vi "Configure Modulation (Frequency).vi"(4 "Peak Deviation (100.00 Hz)":dbl=100.0, 6 "Modulation Frequency (10 Hz)":dbl=10.0, 7 "Enable Frequency Modulation (T:Enable)":bool=TRUE, 8 "error in (no error)":errorcluster, 9 "Modulation Waveform (Sine)":T1(ring), 10 "FM Source (Internal)":enum16{"Internal", "External"}(ring), 11 "VISA resource name":refnum<visa-resource-name>) -> (0 "error out":errorcluster, 3 "VISA resource name out":refnum<visa-resource-name>)   [LabVIEW 2017, in "Keithley 3390.lvlib"]
doc: "Configures and enables frequency modulation (FM). In FM, the frequency of the carrier is varied by the frequency of the modulating waveform. \n\n<B>Note:</B> The carrier waveform shape and parameters are set by the Configure Waveform VI."
uses:
  Keithley 3390.lvlib
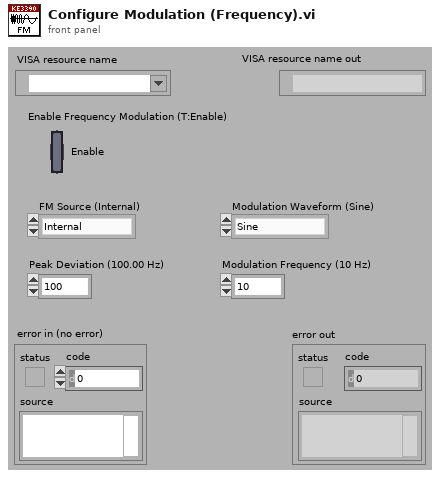
[diagram p1: front panel]
types:
  T1 = enum16{"Sine", "Square", "Ramp", "Negative Ramp", "Triangle", "Noise", "Arbitrary"}
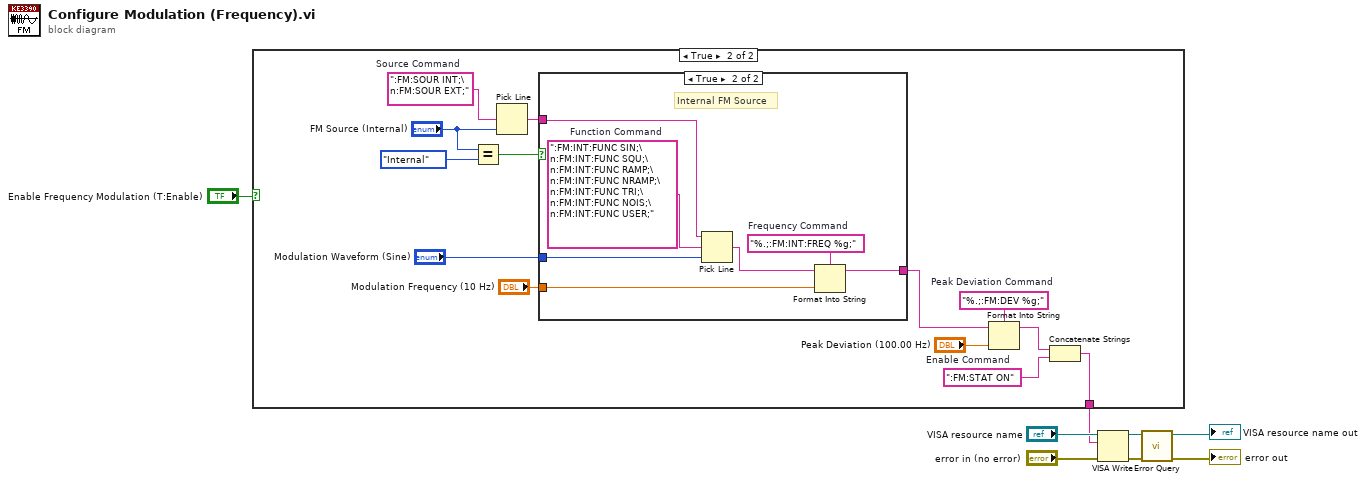
[diagram p0: block diagram]
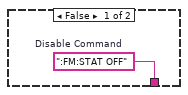
[diagram p2: hidden frame]
diagram:
  n1 = case shown="True" "Enable Frequency Modulation (T:Enable)" {
    tunnel: [w9 w13] -> w6
    frame False {
      w9 = ":FM:STAT OFF"  # Disable Command
    }
    frame True {
      w11 = ":FM:STAT ON"  # Enable Command
      w18 = ":FM:SOUR INT;\n:FM:SOUR EXT;"  # Source Command
      w21 = "%.;:FM:DEV %g;"  # Peak Deviation Command
      n2 = Equal?(x="FM Source (Internal)", y=enum16{"Internal", "External"}."Internal") -> (x = y?=w16:bool)
      n3 = Pick Line(multi-line string=w18, line index="FM Source (Internal)") -> (output string=w15:string)  [unwired: 1 in]
      n4 = case shown="True" w16 {
        tunnel: [w23 w28] -> w20
        tunnel: "Modulation Frequency (10 Hz)" -> [_ w27]
        tunnel: w15 -> [w23 w25]
        tunnel: "Modulation Waveform (Sine)" -> [_ w24]
        frame False {
          # "External FM Source"
        }
        frame True {
          w26 = ":FM:INT:FUNC SIN;\n:FM:INT:FUNC SQU;\n:FM:INT:FUNC RAMP;\n:FM:INT:FUNC NRAMP;\n:FM:INT:FUNC TRI;\n:FM:INT:FUNC NOIS;\n:FM:INT:FUNC USER;"  # Function Command
          w30 = "%.;:FM:INT:FREQ %g;"  # Frequency Command
          # "Internal FM Source"
          n5 = Pick Line(string ("")=w25, multi-line string=w26, line index=w24) -> (output string=w29:string)
          n6 = Format Into String(format string=w30, initial string=w29, w27) -> (resulting string=w28:string)  [unwired: 1 in, 1 out]
        }
      }
      n7 = Format Into String(format string=w21, initial string=w20, "Peak Deviation (100.00 Hz)") -> (resulting string=w12:string)  [unwired: 1 in, 1 out]
      n8 = Concatenate Strings(w12, w11) -> (w13:string)
    }
  }
  n9 = VISA Write(VISA resource name="VISA resource name", write buffer=w6, error in (no error)="error in (no error)") -> (VISA resource name out=w4:refnum<visa-resource-name>, error out=w5:errorcluster)  [unwired: 1 out]
  n10 = call "Error Query.vi"("error in (no error)"=w5, "VISA resource name"=w4) -> ("error out"=→"error out":errorcluster, "VISA resource name out"=→"VISA resource name out":refnum<visa-resource-name>)  [unwired: 6 in, 2 out]
